vi "SwitchedDMM.vi"(4 "DMM ClassName":string="Sim DMM", 5 "Setting":T1={"Resolution (Digits)"=5.5, "Current Source (Amps)"=0.001, "Range"=2.0, "Measurement Type"=enum."4-wire Resistance"} {"Resolution (Digits)" items=["3 1/2"=3.5, "4 1/2"=4.5, "5 1/2"=5.5, "6 1/2"=6.5, "7 1/2"=7.5]; "Current Source (Amps)" items=["1uA"=1e-06, "10uA"=1e-05, "100uA"=0.0001, "1mA"=0.001]}, 6 "DMM Resource":string, 7 "Connection(s)":string="ch49->com3", 8 "error in":errorcluster, 9 "Switch Resource":string, 10 "Switch ClassName":string="Sim Switch", 11 "Base Path":path=path "C:/GitHub/OOP_Submodule EOL/Sequence/CodeModules/HAL/Concrete") -> (0 "error out":errorcluster, 3 "Measurements":dbl=7.500284645380634)   [LabVIEW 2019, in "Wrappers.lvlib"]
uses:
  Wrappers.lvlib
  BSM OOP/Sequence/CodeModules/Hardware Abstraction/Harware Abstraction/Switch/Switch.lvclass
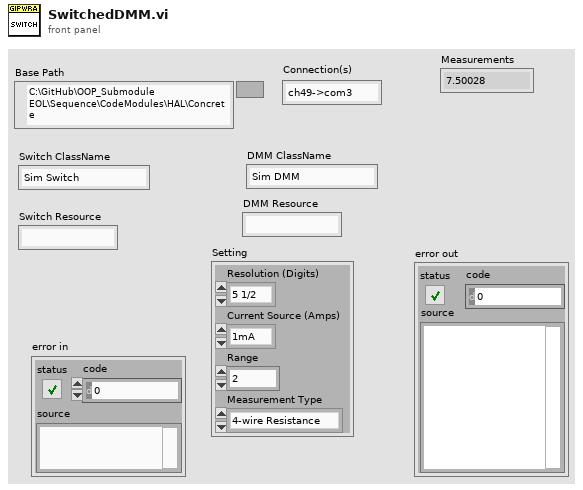
[diagram p1: front panel]
types:
  T1 = cluster{"Resolution (Digits)":dbl, "Current Source (Amps)":dbl, "Range":dbl, "Measurement Type":enum16{"DC Volts", "AC Volts", "DC Current", "AC Current", "2-wire Resistance", "4-wire Resistance", "Diode", "Frequency", "Period", "AC Volts DC Coupled", "Capacitance", "Inductance", "Temperature"}}
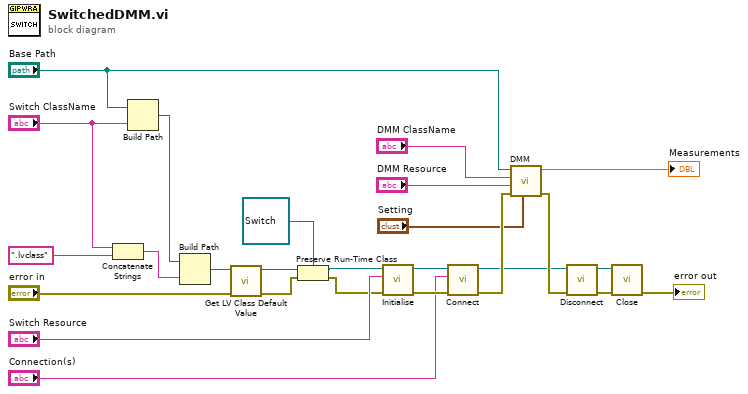
[diagram p0: block diagram]
diagram:
  n1 = Concatenate Strings("Switch ClassName", ".lvclass" ("string")) -> (w2:string)
  n2 = Build Path(base path="Base Path", name or relative path="Switch ClassName") -> (appended path=w4:path)
  n3 = Build Path(base path=w4, name or relative path=w2) -> (appended path=w24:path)
  n4 = call <vilib>:"Get LV Class Default Value.vi"("error in (no error)"="error in", "class path"=w24) -> ("error out"=w23:errorcluster, "object"=w25:refnum<class>)  [unwired: 8 in]
  n5 = Preserve Run-Time Class(object in=w25, error in=w23, 2:refnum<class "Switch.lvclass"> refnum ("Hardware Abstration.lvlib:Switch.lvclass")) -> (object out=w21:refnum<class "Switch.lvclass">, error out=w20:errorcluster)
  n6 = call-dynamic "Initialise.vi"("error in (no error)"=w20, "Instrument Ref"="Switch Resource", "Instrument in"=w21) -> ("error out"=w18:errorcluster, "Instrument out"=w17:refnum<class "Switch.lvclass">)  [unwired: 7 in]
  n7 = call-dynamic "Connect.vi"("error in (no error)"=w18, "Channel(s)"="Connection(s)", "Switch in"=w17) -> ("error out"=w13:errorcluster, "Switch out"=w11:refnum<class "Switch.lvclass">)  [unwired: 7 in]
  n8 = call "DMM.vi"("Setting"="Setting", "error in"=w13, "DMM Ref"="DMM Resource", "DMM Class"="DMM ClassName", "Base Path"="Base Path") -> ("error out"=w12:errorcluster, "Measurements"=→"Measurements":dbl)  [unwired: 5 in]
  n9 = call-dynamic "Disconnect.vi"("error in (no error)"=w12, "Switch in"=w11) -> ("error out"=w16:errorcluster, "Switch out"=w15:refnum<class "Switch.lvclass">)  [unwired: 8 in]
  n10 = call-dynamic "Close.vi"("error in (no error)"=w16, "Instrument in"=w15) -> ("error out"=→"error out":errorcluster)  [unwired: 8 in, 1 out]
